vi "23384_Davis_Poku_Amankwa_Amankwa.DavisPoku.MNE1201.3.1_348255_705380801.vi"() -> ()   [LabVIEW 2018]
panel:
  out "Monthly pay at the end of the month of 30days in dollars":dbl
  # "1$=100pennies"
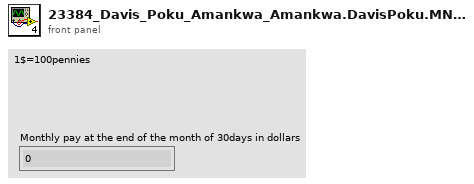
[diagram p1: front panel]
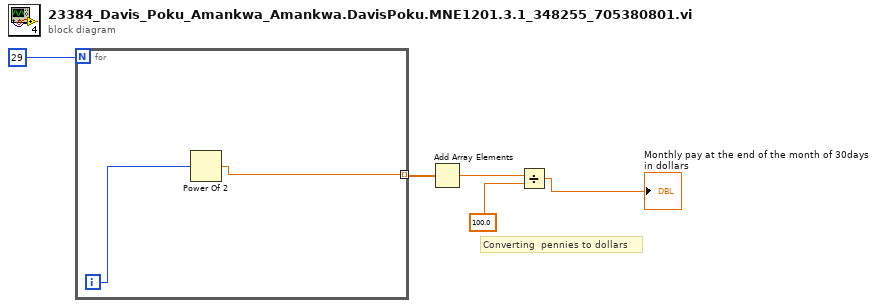
[diagram p0: block diagram]
diagram:
  # "Converting  pennies to dollars"
  n1 = for {
    N: 29 -> [_]
    tunnel: [w6] -> w4 mode=indexing
    i -> [w7]
    n2 = Power Of 2(x=w7) -> (2^x=w6:dbl)
  }
  n3 = Add Array Elements(numeric array=w4) -> (sum=w3:dbl)
  n4 = Divide(x=w3, y=100.0) -> (x/y=→"Monthly pay at the end of the month of 30days in dollars":dbl)
